vi "String to SingleFloat (Scalar).vi"(10 "Value (String)":string) -> (1 "Rest of string":string, 2 "Value (Single)":sgl, 3 "offset past number":i32)   [LabVIEW 2013, in "OpenScalar.lvlib"]
uses:
  OpenScalar.lvlib
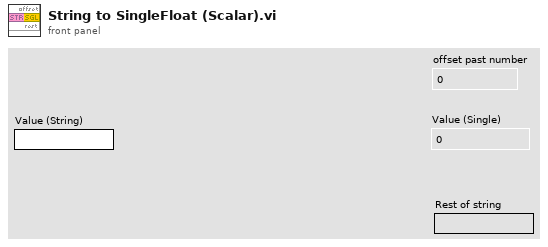
[diagram p1: front panel]
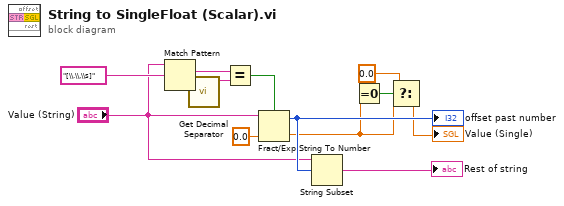
[diagram p0: block diagram]
diagram:
  n1 = Match Pattern(string="Value (String)", regular expression="[\\.\\,\\s]") -> (match substring=w10:string)  [unwired: 1 in, 3 out]
  n2 = call "Get Decimal Separator.vi"() -> ("System Decimal separator"=w8:string)  [unwired: 11 in]
  n3 = Equal?(x=w10, y=w8) -> (x = y?=w9:bool)
  n4 = Fract/Exp String To Number(use system decimal point (T)=w9, string="Value (String)", default (0 dbl)=sgl 0.0 ("default (0 DBL)")) -> (offset past number=w7:i32, number=w3:sgl)  [unwired: 1 in]
  "offset past number" <- w7
  n5 = String Subset(string="Value (String)", offset (0)=w7) -> (substring=→"Rest of string":string)  [unwired: 1 in]
  n6 = Equal To 0?(x=w3) -> (x = 0?=w4:bool)
  n7 = Select(t=sgl 0.0, s=w4, f=w3) -> (s? t:f=→"Value (Single)":sgl)
